vi "Do.vi"(8 "error in (no error)":errorcluster, 10 "Actor in":refnum<class "Actor.lvclass">, 11 "Register PVs Msg":refnum<class "Register PVs Msg.lvclass">) -> (0 "error out":errorcluster, 2 "Actor out":refnum<class "Actor.lvclass">)   [LabVIEW 2016, in "CS++PVProxy.lvlib" / "Register PVs Msg.lvclass"]
doc: "(<B>Filename</B>: Actor Framework.lvlib:Message.lvclass:Do.vi)\n\nDefines what a message does when it is received by an actor. Generally, a message instructs an actor to invoke one of its methods. By default, this method does nothing. A child class must override it to define behavior. Create a child class by using the Actor Framework Message Maker dialog box."
uses:
  Register PVs Msg.lvclass
  <vilib>/ActorFramework/Actor/Actor.lvclass
  C:/User/Brand/LVP/CSPP/Packages/CSPP_Core/Actors/CS++PVMonitor Messages/CS++PVUpdate Msg/CS++PVUpdate Msg.lvclass
  CS++PVProxy/CS++PVProxy.lvclass
  C:/Program Files (x86)/National Instruments/LabVIEW 2016/vi.lib/ActorFramework/Actor/Actor.lvclass
  CS++PVMonitor Messages/CS++PVUpdate Msg/CS++PVUpdate Msg.lvclass/CS++PVUpdate Msg.ctl
  Classes/CS++ProcessVariables/ProcessVariable/PV.lvclass/PV.ctl
  Register PVs Msg.lvclass/Register PVs Msg.ctl
  Classes/CS++ProcessVariables/ProcessVariable/PV.lvclass
  CS++PVMonitor Messages/CS++PVUpdate Msg/CS++PVUpdate Msg.lvclass
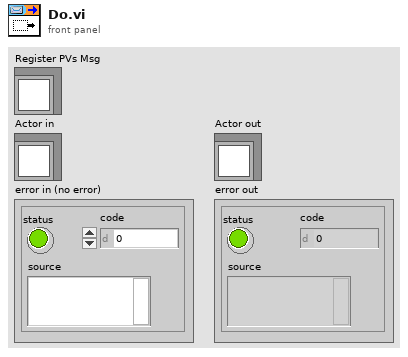
[diagram p1: front panel]
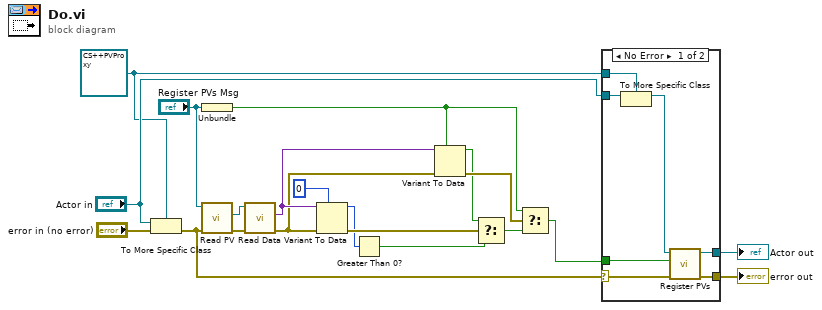
[diagram p0: block diagram]
diagram:
  w16 = refnum<class "CS++PVProxy.lvclass"> refnum ("Actor in")
  n1 = To More Specific Class(target class=w16, reference="Actor in", error in="error in (no error)") -> (error out=w14:errorcluster)  [unwired: 1 out]
  n2 = Unbundle ("Pre-Unbundler")("Register PVs Msg") -> (w3:bool)
  n3 = call "Read PV.vi"("error in (no error)"=w14, "CS++PVUpdate Msg in"="Register PVs Msg") -> ("error out"=w13:errorcluster, "PV"=w11:refnum<class "PV.lvclass">)  [unwired: 7 in, 1 out]
  n4 = call "Read Data.vi"("error in (no error)"=w13, "PV in"=w11) -> ("error out"=w8:errorcluster, "Data"=w9:variant)  [unwired: 7 in, 1 out]
  n5 = Variant To Data ("I16-Conversion")(error in=w8, type=i16 0 ("I16-Conversion-Constant"), Variant=w9) -> (data=w4:i16, error out=w7:errorcluster)
  n6 = Greater Than 0? ("I16-Comp0")(x=w4) -> (x > 0?=w2:bool)
  n7 = Variant To Data(error in=w8, type=w3, Variant=w9) -> (data=w6:bool, error out=w12:errorcluster)
  n8 = Select ("I16-Select")(t=w6, s=w7, f=w2) -> (s? t:f=w5:bool)
  n9 = Select ("MainSelect")(t=w3, s=w12, f=w5) -> (s? t:f=w1:bool)
  n10 = case shown="No Error" w14 {
    selector: w14 -> [w25 w29]
    tunnel: [w27 w29] -> w19
    tunnel: [w26 w28] -> w18
    tunnel: "Actor in" -> [w24 w28]
    tunnel: w16 -> [w23 _]
    tunnel: w1 -> [w21 _]
    frame No Error {
      n11 = To More Specific Class(target class=w23, reference=w24) -> (specific class reference=w22:refnum<class "CS++PVProxy.lvclass">)  [unwired: 1 in, 1 out]
      n12 = call "Register PVs.vi"("error in (no error)"=w25, "Activate?"=w21, "CS++PVProxy in"=w22) -> ("error out"=w27:errorcluster, "CS++PVProxy out"=w26:refnum<class "CS++PVProxy.lvclass">)  [unwired: 7 in]
    }
    frame Error {
    }
  }
  "error out" <- w19
  "Actor out" <- w18
